vi "Format Table Pretty.vi"(9 "Program":u16, 10 "Program 2":refnum<vi>, 11 "Programs in":refnum<class "Programs.lvclass">) -> (3 "Array":string[][](array[string]))   [LabVIEW 2025]
uses:
  Classes/Programs/Programs.lvclass
  <vilib>/Analysis/baseanly.llb/Mean (DBL).vi
  <vilib>/Analysis/NI_AALBase.lvlib
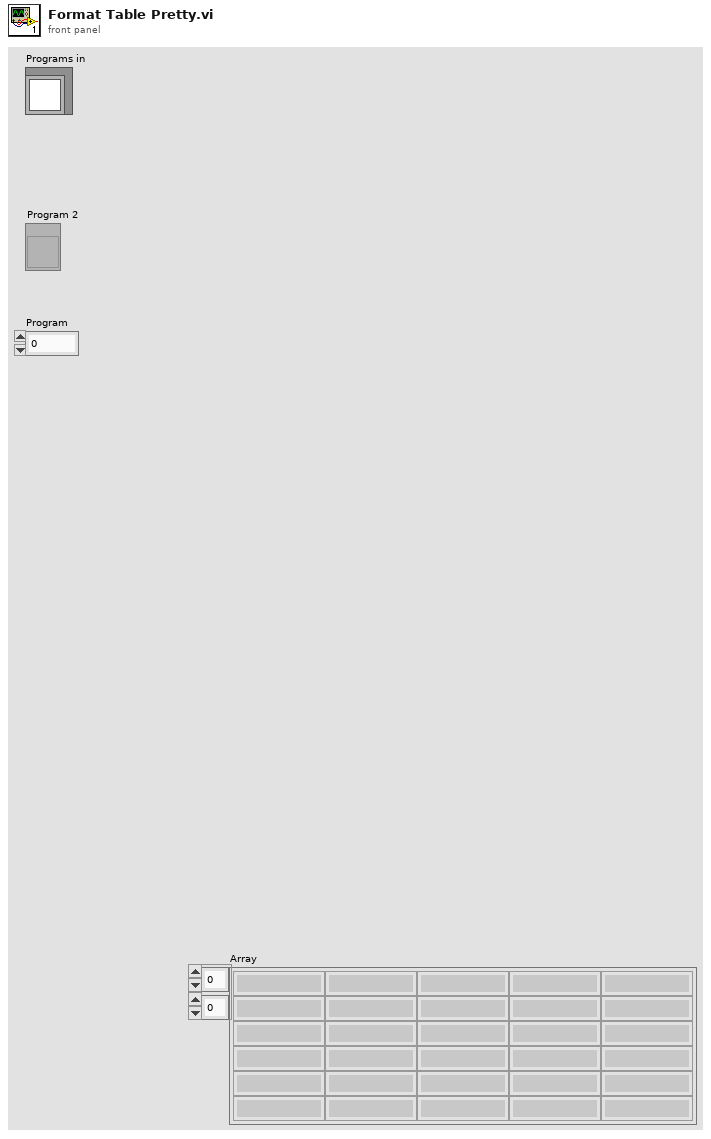
[diagram p1: front panel]
types:
  T1 = typedef "sequence array.ctl" = T2[]
  T2 = typedef "step cluster.ctl" = cluster{"Action":T3, "Angle Min [°]":dbl, "Angle Max [°]":dbl, "Torque Min [oz-in]":dbl, "Torque Max [oz-in]":dbl}
  T3 = typedef "action enum.ctl" = enum16{"Start", "Angle", "Return to Home", "End"}
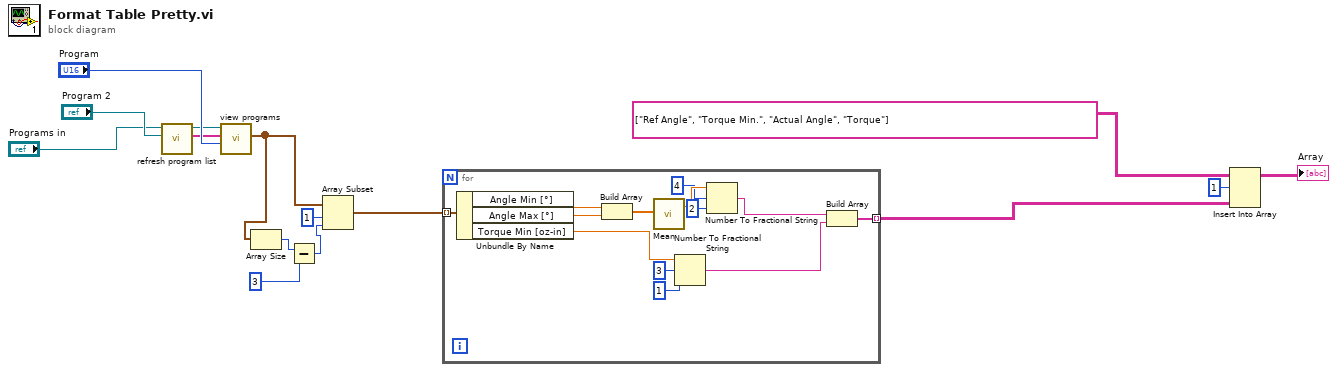
[diagram p0: block diagram]
diagram:
  n1 = call-dynamic "refresh program list.vi"("reference"="Program 2", "Programs in"="Programs in") -> ("Program List"=w13:string[], "Programs out"=w14:refnum<class "Programs.lvclass">)  [unwired: 7 in, 1 out]
  n2 = call-dynamic "view programs.vi"("Program"="Program", "Program List"=w13, "Programs in"=w14) -> ("Data out"=w9:T1)  [unwired: 6 in, 2 out]
  n3 = Array Size(array=w9) -> (size(s)=w8:i32)
  n4 = Subtract(x=w8, y=3) -> (x-y=w6:i32)
  n5 = Array Subset(array=w9, index=1, length=w6) -> (w5:T1)
  n6 = for {
    tunnel: w5 -> [w28] mode=indexing
    tunnel: [w24] -> w3 mode=indexing
    n7 = Unbundle By Name(w28) -> ("Angle Min [°]"=w26:dbl, "Angle Max [°]"=w27:dbl, "Torque Min [oz-in]"=w19:dbl)
    n8 = Build Array(w26, w27) -> (w25:dbl[])
    n9 = call-poly <vilib>:"Mean.vi"("X"=w25) -> ("mean"=w23:dbl)  [unwired: 1 out]
    n10 = Number To Fractional String(number=w19, width (-)=i16 3, precision (6)=i16 1) -> (F-format string=w18:string)  [unwired: 1 in]
    n11 = Number To Fractional String(number=w23, width (-)=i16 4, precision (6)=i16 2) -> (F-format string=w20:string)  [unwired: 1 in]
    n12 = Build Array(w20, w18) -> (w24:string[])
  }
  n13 = Insert Into Array(array=string[][] [["Ref Angle", "Torque Min.", "Actual Angle", "Torque"]], index (row)=1, new element=w3) -> (→"Array":string[][])  [unwired: 1 in]
